vi "thcd_set_uom.vi"(5 "thcd_delay":u32=500, 6 "err_in":errorcluster, 7 "thcd_val":T1, 8 "thcd_ch":T2, 9 "thcd_visa":refnum<visa-resource-name>) -> (0 "err_out":errorcluster, 1 "thcd_st":bool, 2 "thcd_res_msg":string, 3 "thcd_visa":refnum<visa-resource-name>)   [LabVIEW 2020, in "1039_mod.lvlib"]
uses:
  1039_mod/1039_mod.lvlib
  thcd_controls/ctrl_chn_thcd.ctl
  thcd_controls/ctrl_uom_thcd.ctl
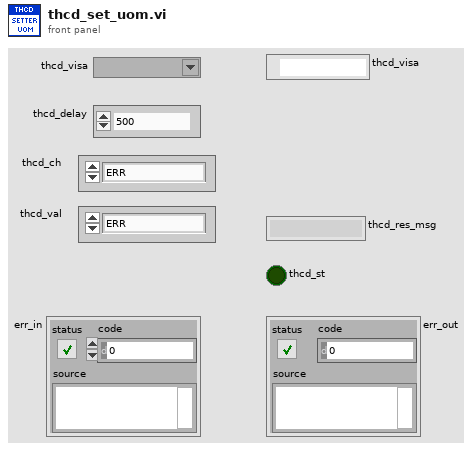
[diagram p1: front panel]
types:
  T1 = typedef "ctrl_uom_thcd.ctl" = enum16{"ERR", "SCCM", "SLM", "%", "V", "MV", "CNT", "NLM", "SLS", "NLS", "SLH", "NLH", "SMLM", "NMLM", "SMLS", "NMLS", "SMLH", "NMLH", "NCCM", "SCCS", "NCCS", "SCCH", "NCCH", "SCFM", "NCFM", "SCFS", "NCFS", "SCFH", "NCFH", "SCMM", "NCMM", "SCMS", "NCMS", "SCMH", "NCMH", "SCIM", "NCIM", "SCIS", "NCIS", "SCIH", "NCIH", "LBM", "LBS", "LBH", "KgM", "KgS", "KgH", "GRM", "GMS", "GRH", "MolM", "MolS", "MolH", "KMolM", "KMolS", "KMolH", "W", "BPS", "Sec", "Min", "Hrs", "WH", "Torr", "Bar", "Pa", "inH2O", "PSIA", "PSIG"}
  T2 = typedef "ctrl_chn_thcd.ctl" = enum8{"ERR", "1", "2", "3", "4"}
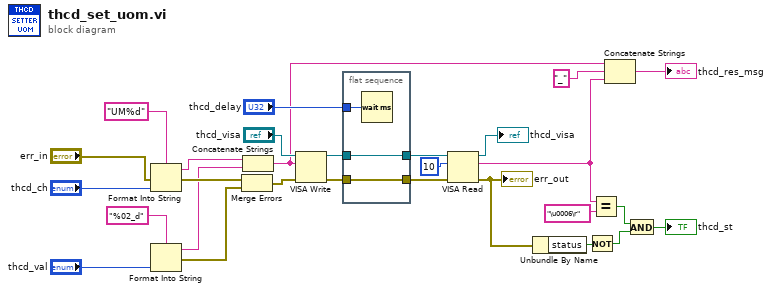
[diagram p0: block diagram]
diagram:
  n1 = Format Into String(format string="UM%d", error in="err_in", "thcd_ch") -> (resulting string=w19:string, error out=w18:errorcluster)  [unwired: 1 in]
  n2 = Format Into String(format string="%02_d", "thcd_val") -> (resulting string=w15:string, error out=w16:errorcluster)  [unwired: 2 in]
  n3 = Merge Errors(w18, w16) -> (w17:errorcluster)
  n4 = Concatenate Strings(w19, w15) -> (w3:string)
  n5 = VISA Write(VISA resource name="thcd_visa", write buffer=w3, error in (no error)=w17) -> (VISA resource name out=w27:refnum<visa-resource-name>, error out=w28:errorcluster)  [unwired: 1 out]
  n6 = flat-sequence {
    tunnel: w28 -> [w30]
    tunnel: [w30] -> w7
    tunnel: w27 -> [w29]
    tunnel: [w29] -> w11
    tunnel: "thcd_delay" -> [w31]
    frame #0 {
      n7 = Wait (ms)(milliseconds to wait=w31) -> ()  [unwired: 1 out]
    }
  }
  n8 = VISA Read(VISA resource name=w11, byte count=u32 10, error in (no error)=w7) -> (VISA resource name out=→"thcd_visa":refnum<visa-resource-name>, read buffer=w1:string, error out=w6:errorcluster)  [unwired: 1 out]
  "err_out" <- w6
  n9 = Unbundle By Name(w6) -> ("status"=w20:bool)
  n10 = Not(x=w20) -> (.not. x?=w9:bool)
  n11 = Equal?(x=w1, y="\u0006\r") -> (x = y?=w10:bool)
  n12 = Concatenate Strings(w3, "_", w1) -> (→"thcd_res_msg":string)
  n13 = And(x=w10, y=w9) -> (x .and. y?=→"thcd_st":bool)
